vi "Update Data.vi"(8 "error in (no error)":errorcluster, 9 "data":waveform(dbl)[](array[waveform]), 10 "Channel Names":string[](array[string]), 11 "[V]Waveform Display in":refnum<class "[V]Waveform Display.lvclass">) -> (0 "error out":errorcluster, 3 "[V]Waveform Display out":refnum<class "[V]Waveform Display.lvclass">)   [LabVIEW 2020, in "[V]Waveform Display.lvlib" / "[V]Waveform Display.lvclass"]
uses:
  [V]Waveform Display.lvclass
  [V]Waveform Display.lvclass/[V]Waveform Display.ctl
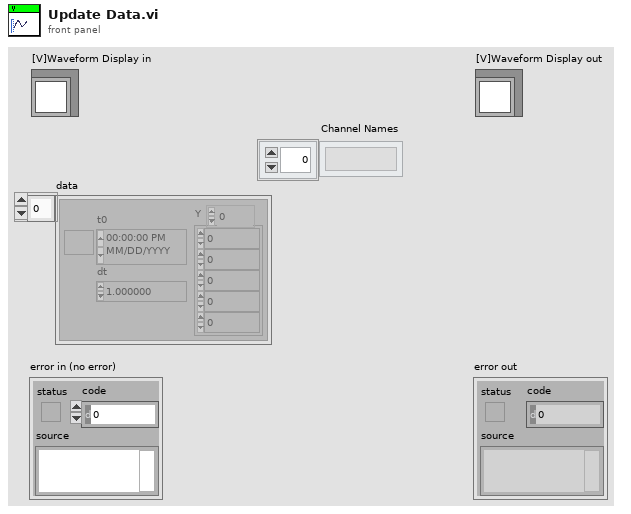
[diagram p1: front panel]
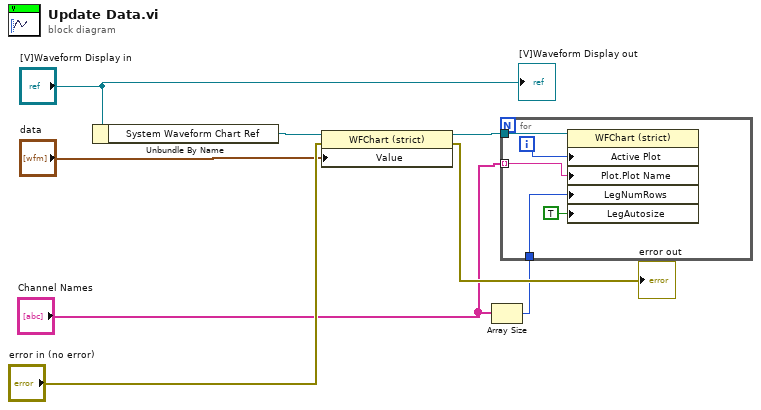
[diagram p0: block diagram]
diagram:
  n1 = Unbundle By Name("[V]Waveform Display in") -> ("System Waveform Chart Ref"=w7:refnum<vi>)
  n2 = property class="WFChart (strict)"(reference=w7, error in="error in (no error)", "Value"="data") -> (reference out=w4:refnum<vi>, error out=→"error out":errorcluster)
  n3 = Array Size(array="Channel Names") -> (size(s)=w1:i32)
  n4 = for {
    tunnel: w4 -> [w13]
    tunnel: "Channel Names" -> [w11] mode=indexing
    tunnel: w1 -> [w9]
    i -> [w12]
    n5 = property class="WFChart (strict)"(reference=w13, "Active Plot"=w12, "Plot.Plot Name"=w11, "LegNumRows"=w9, "LegAutosize"=TRUE ("Legend:Autosize")) -> ()  [unwired: 1 in, 2 out]
  }
  "[V]Waveform Display out" <- "[V]Waveform Display in"
